vi "#197-Caller.vi"() -> ()   [LabVIEW 2014]
uses:
  user.lib/_NEVSTOP/Communicable State Machine(CSM)/_Support/Priority Queue/Priority Queue.lvclass/Priority Queue.ctl
  user.lib/_NEVSTOP/Communicable State Machine(CSM)/_Support/Process/CSMP-Sync Call.vi
  user.lib/_NEVSTOP/Communicable State Machine(CSM)/Utility/uuid.vi
  user.lib/_NEVSTOP/Communicable State Machine(CSM)/Utility/Trim Both Whitespace.vi
  user.lib/_NEVSTOP/Communicable State Machine(CSM)/_Support/Process/CSMP-Async Call.vi
  user.lib/_NEVSTOP/Communicable State Machine(CSM)/_Support/CSMQ/_CSMObj-Message Check.vi
  user.lib/_NEVSTOP/Communicable State Machine(CSM)/_Support/CSMQ/_CSMObj-Enqueue Cross-Module Message.vi
  user.lib/_NEVSTOP/Communicable State Machine(CSM)/_Support/CSMQ/_CSMOFGV Get.vi
  user.lib/_NEVSTOP/Communicable State Machine(CSM)/_Support/Priority Queue/Enqueue Element.vi
  user.lib/_NEVSTOP/Communicable State Machine(CSM)/Utility/Build Error Cluster.vi
  user.lib/_NEVSTOP/Communicable State Machine(CSM)/_Support/CSMQ/_CSMOFGV.vi
  user.lib/_NEVSTOP/Communicable State Machine(CSM)/Communicable State Machine.lvlib
panel:
  out "Diff Timer(s)":dbl format="%.6f"
  out "error IO":errorcluster
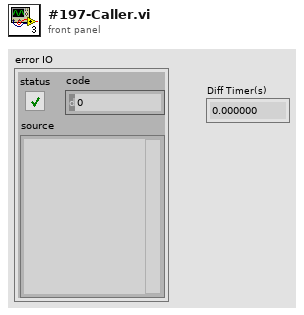
[diagram p1: front panel]
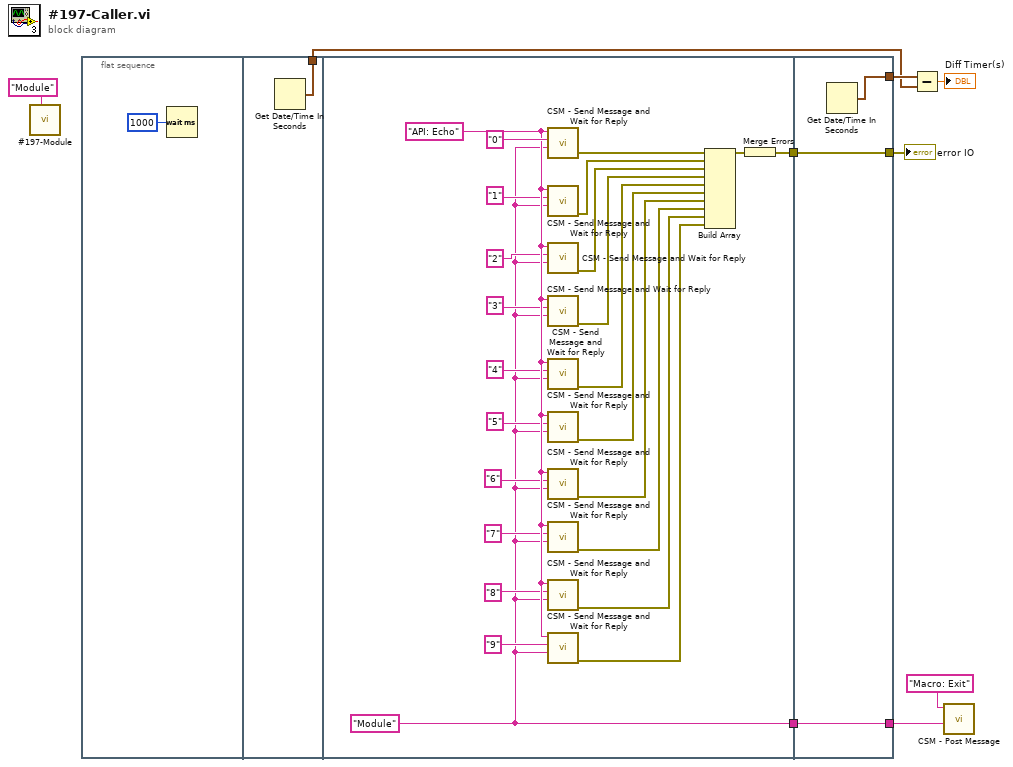
[diagram p0: block diagram]
diagram:
  n1 = call "#197-Module.vi"("Name(\"\" to use uuid)"="Module" ("Name(\"\" to use uuid)")) -> ()  [unwired: 11 in]
  n2 = flat-sequence {
    tunnel: [w11] -> w2
    tunnel: [w12] -> w6
    tunnel: [w22] -> w5
    tunnel: [w37] -> w7
    tunnel: [w38] -> w8
    tunnel: w6 -> [w38]
    tunnel: w5 -> [w37]
    tunnel: [w36] -> w4
    frame #0 {
      n3 = Wait (ms)(milliseconds to wait=u32 1000) -> ()  [unwired: 1 out]
    }
    frame #1 {
      n4 = Get Date/Time In Seconds() -> (seconds since 1Jan1904=w11:timestamp)
    }
    frame #2 {
      w34 = "API: Echo" ("State")
      w22 = "Module" ("Name(\"\" to use uuid)")
      n5 = call "CSM - Send Message and Wait for Reply.vi"("Target Module"=w22, "Arguments (\"\")"="0" ("Arguments (\"\")"), "State"=w34) -> ("error out"=w24:errorcluster)  [unwired: 6 in, 2 out]
      n6 = call "CSM - Send Message and Wait for Reply.vi"("Target Module"=w22, "Arguments (\"\")"="1" ("Arguments (\"\")"), "State"=w34) -> ("error out"=w21:errorcluster)  [unwired: 6 in, 2 out]
      n7 = call "CSM - Send Message and Wait for Reply.vi"("Target Module"=w22, "Arguments (\"\")"="2" ("Arguments (\"\")"), "State"=w34) -> ("error out"=w20:errorcluster)  [unwired: 6 in, 2 out]
      n8 = call "CSM - Send Message and Wait for Reply.vi"("Target Module"=w22, "Arguments (\"\")"="3" ("Arguments (\"\")"), "State"=w34) -> ("error out"=w19:errorcluster)  [unwired: 6 in, 2 out]
      n9 = call "CSM - Send Message and Wait for Reply.vi"("Target Module"=w22, "Arguments (\"\")"="4" ("Arguments (\"\")"), "State"=w34) -> ("error out"=w18:errorcluster)  [unwired: 6 in, 2 out]
      n10 = call "CSM - Send Message and Wait for Reply.vi"("Target Module"=w22, "Arguments (\"\")"="5" ("Arguments (\"\")"), "State"=w34) -> ("error out"=w17:errorcluster)  [unwired: 6 in, 2 out]
      n11 = call "CSM - Send Message and Wait for Reply.vi"("Target Module"=w22, "Arguments (\"\")"="6" ("Arguments (\"\")"), "State"=w34) -> ("error out"=w16:errorcluster)  [unwired: 6 in, 2 out]
      n12 = call "CSM - Send Message and Wait for Reply.vi"("Target Module"=w22, "Arguments (\"\")"="7" ("Arguments (\"\")"), "State"=w34) -> ("error out"=w15:errorcluster)  [unwired: 6 in, 2 out]
      n13 = call "CSM - Send Message and Wait for Reply.vi"("Target Module"=w22, "Arguments (\"\")"="8" ("Arguments (\"\")"), "State"=w34) -> ("error out"=w14:errorcluster)  [unwired: 6 in, 2 out]
      n14 = call "CSM - Send Message and Wait for Reply.vi"("Target Module"=w22, "Arguments (\"\")"="9" ("Arguments (\"\")"), "State"=w34) -> ("error out"=w13:errorcluster)  [unwired: 6 in, 2 out]
      n15 = Build Array(w24, w21, w20, w19, w18, w17, w16, w15, w14, w13) -> (w23:errorcluster[])
      n16 = Merge Errors(w23) -> (w12:errorcluster)
    }
    frame #3 {
      n17 = Get Date/Time In Seconds() -> (seconds since 1Jan1904=w36:timestamp)
    }
  }
  n18 = Subtract(x=w4, y=w2) -> (x-y=→"Diff Timer(s)":dbl)
  n19 = call "CSM - Post Message.vi"("Target Module"=w7, "State"="Macro: Exit") -> ()  [unwired: 9 in, 1 out]
  "error IO" <- w8
